vi "Event Handler.vi"(8 "error in (no error)":errorcluster, 10 "Stop Event Hander":refnum<user-event>, 11 "LargeScrollbar in":refnum<class "LargeScrollbar.lvclass">) -> (0 "error out":errorcluster)   [LabVIEW 2015, in "LargeScrollbar.lvclass"]
doc: "The <b>Event Handler VI</b> is a dynamic dispatch VI that should be overwritten if events are needed to create the enhanced QControl. \n\nBy inheriting from the main Control.lvclass the overwritten <b>Event Handler VI</b> will be launched asynchronously in the initialization of the QControl.\n<b> </b> <b> </b>\n©2016 Q Software Innovations, LLC (QSI)\nwritten by Quentin Alldredge\nproduced in LabVIEW 2015\n\nsupport@qsoftwareinnovations.com\nwww.qsoftwareinnovations.com\n\nAll rights reserved.\n\nRedistribution and use in source and binary forms, with or without modification, are permitted provided that the following conditions are met:\n\n * Redistributions of source code must retain the above copyright notice, this list of conditions and the following disclaimer.\n * Redistributions in binary form must reproduce the above copyright notice, this list of conditions and the following disclaimer in the documentation and/or other materials provided with the distribution.\n * Neither the name of Q Software Innovations, LLC. nor the names of its contributors may be used to endorse or promote products derived from this software without specific prior written permission.\n\nTHIS SOFTWARE IS PROVIDED BY THE COPYRIGHT HOLDERS AND CONTRIBUTORS \"AS IS\" AND ANY EXPRESS OR IMPLIED WARRANTIES, INCLUDING, BUT NOT LIMITED TO, THE IMPLIED WARRANTIES OF MERCHANTABILITY AND FITNESS FOR A PARTICULAR PURPOSE ARE DISCLAIMED. IN NO EVENT SHALL THE COPYRIGHT OWNER OR CONTRIBUTORS BE LIABLE FOR ANY DIRECT, INDIRECT, INCIDENTAL, SPECIAL, EXEMPLARY, OR CONSEQUENTIAL DAMAGES (INCLUDING, BUT NOT LIMITED TO, PROCUREMENT OF SUBSTITUTE GOODS OR SERVICES; LOSS OF USE, DATA, OR PROFITS; OR BUSINESS INTERRUPTION) HOWEVER CAUSED AND ON ANY THEORY OF LIABILITY, WHETHER IN CONTRACT, STRICT LIABILITY, OR TORT (INCLUDING NEGLIGENCE OR OTHERWISE) ARISING IN ANY WAY OUT OF THE USE OF THIS SOFTWARE, EVEN IF ADVISED OF THE POSSIBILITY OF SUCH DAMAGE."
uses:
  LargeScrollbar.lvclass
  LargeScrollbar.lvclass/LargeScrollbar.ctl
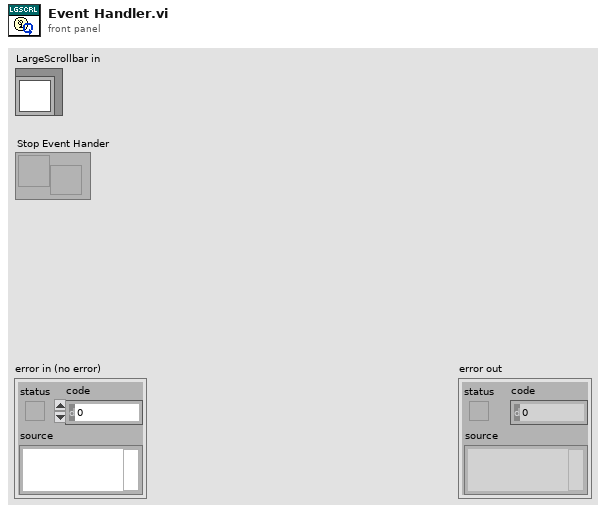
[diagram p1: front panel]
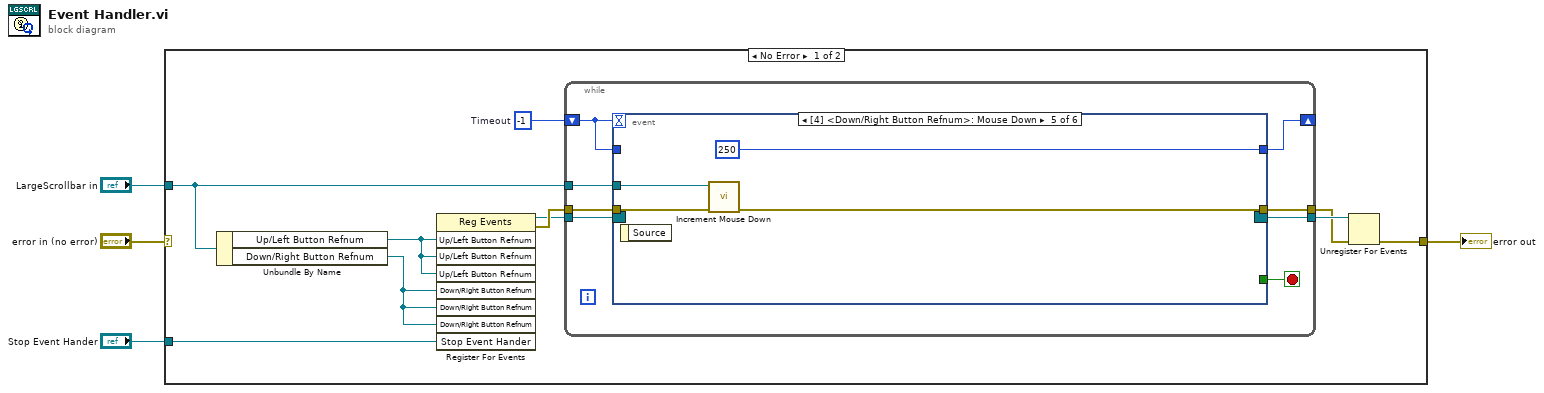
[diagram p0: block diagram]
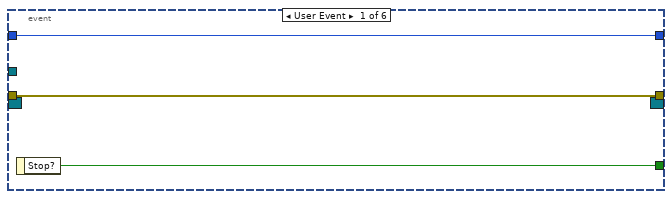
[diagram p2: hidden frame]
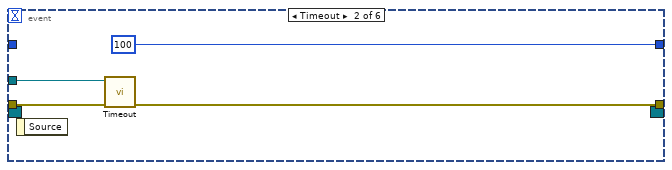
[diagram p3: hidden frame]
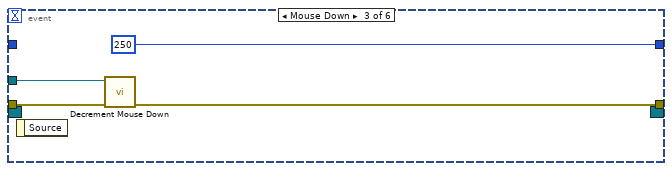
[diagram p4: hidden frame]
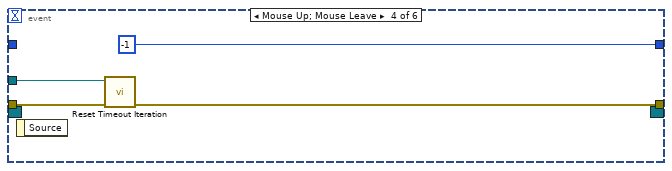
[diagram p5: hidden frame]
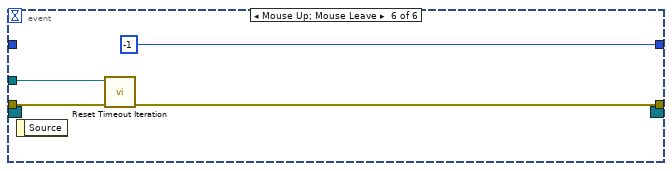
[diagram p6: hidden frame]
diagram:
  n1 = case shown="No Error" "error in (no error)" {
    selector: "error in (no error)" -> [_ w46]
    tunnel: [w11 w46] -> w3
    tunnel: "LargeScrollbar in" -> [w14 _]
    tunnel: "Stop Event Hander" -> [w5 _]
    frame No Error {
      w12 = -1  # Timeout
      n2 = Unbundle By Name(w14) -> ("Up/Left Button Refnum"=w8:refnum<vi>, "Down/Right Button Refnum"=w7:refnum<vi>)
      n3 = register-events(w8, w8, w8, w7, w7, w7, w5) -> (reference out=w6:refnum<event-registration>, error out=w13:errorcluster)  [unwired: 2 in]
      n4 = while {
        tunnel: w6 -> [w15]
        tunnel: w13 -> [w20]
        shift-right: [w19] -> _
        shift-left: w12 -> [w16]
        tunnel: [w18] -> w10
        tunnel: [w17] -> w9
        tunnel: w14 -> [w22]
        stop <- w21 stop-if-true
        n5 = event shown="[4] <Down/Right Button Refnum>: Mouse Down" {
          selector: w15 -> [_ _ _ _ _ _]
          dyn-events: [_ _ _ _ _ _] -> w18
          timeout: w16 -> [_ _ _ _ _ _]
          tunnel: w22 -> [_ w27 w31 w36 w39 w42]
          tunnel: [w25 _ _ _ _ _] -> w21
          tunnel: w20 -> [w24 w29 w30 w35 w41 w44]
          tunnel: [w23 100 250 -1 250 -1] -> w19
          tunnel: [w24 w28 w32 w34 w38 w43] -> w17
          tunnel: w16 -> [w23 _ _ _ _ _]
          event User Event {
            n6 = event-data() -> ("Stop?"=w25:bool)  [unwired: 1 in]
          }
          event Timeout {
            n7 = event-data() -> ()  [unwired: 1 in, 1 out]
            n8 = call "Timeout.vi"("error in (no error)"=w29, "LargeScrollbar in"=w27) -> ("error out"=w28:errorcluster)  [unwired: 9 in]
          }
          event Mouse Down {
            n9 = event-data() -> ()  [unwired: 1 in, 1 out]
            n10 = call "Decrement Mouse Down.vi"("error in (no error)"=w30, "LargeScrollbar in"=w31) -> ("error out"=w32:errorcluster)  [unwired: 9 in]
          }
          event Mouse Up; Mouse Leave {
            n11 = event-data() -> ()  [unwired: 1 in, 1 out]
            n12 = call "Reset Timeout Iteration.vi"("error in (no error)"=w35, "LargeScrollbar in"=w36) -> ("error out"=w34:errorcluster)  [unwired: 8 in, 1 out]
          }
          event Mouse Down {
            n13 = event-data() -> ()  [unwired: 1 in, 1 out]
            n14 = call "Increment Mouse Down.vi"("error in (no error)"=w41, "LargeScrollbar in"=w39) -> ("error out"=w38:errorcluster)  [unwired: 9 in]
          }
          event Mouse Up; Mouse Leave {
            n15 = event-data() -> ()  [unwired: 1 in, 1 out]
            n16 = call "Reset Timeout Iteration.vi"("error in (no error)"=w44, "LargeScrollbar in"=w42) -> ("error out"=w43:errorcluster)  [unwired: 8 in, 1 out]
          }
        }
      }
      n17 = Unregister For Events(event registration refnum=w10, error in=w9) -> (error out=w11:errorcluster)
    }
    frame Error {
    }
  }
  "error out" <- w3
